vi "Init Name Description.vi"(8 "error in (no error)":errorcluster, 9 "Description":refnum<vi>, 10 "Name":refnum<vi>, 11 "Node Ptr":T1 format="%.0x") -> (0 "error out":errorcluster, 3 "Node Ptr out":T1=18446744073709551615 format="%.0x")   [LabVIEW 2014, in "SLSC configuration System Explorer.lvlib"]
uses:
  SLSC configuration System Explorer.lvlib
  <vilib>/NI Veristand/Custom Device API/Custom Device Item Ref.ctl
  <vilib>/NI Veristand/Custom Device API/Custom Device API.lvlib
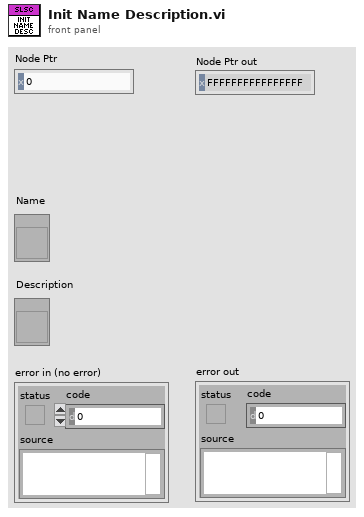
[diagram p1: front panel]
types:
  T1 = typedef "Custom Device API.lvlib/Custom Device Item Ref.ctl" = u64
  T2 = typedef "Custom Device API.lvlib/Custom Device Item Info.ctl" = cluster{"Name":string, "Is Channel":bool, "GUID":string, "Is Waveform":bool}
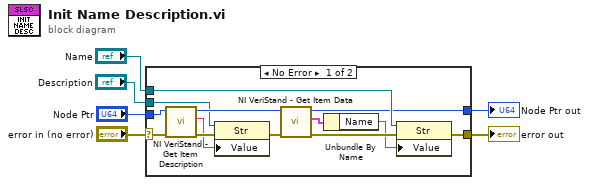
[diagram p0: block diagram]
diagram:
  n1 = case shown="No Error" "error in (no error)" {
    selector: "error in (no error)" -> [w9 w21]
    tunnel: "Node Ptr" -> [w10 w20]
    tunnel: [w7 w20] -> w1
    tunnel: [w8 w21] -> w2
    tunnel: "Description" -> [w12 _]
    tunnel: "Name" -> [w11 _]
    frame No Error {
      n2 = call <vilib>:"NI VeriStand - Get Item Description.vi"("error in (no error)"=w9, "Item Ref in"=w10) -> ("error out"=w19:errorcluster, "Description"=w18:string, "Item Ref out"=w13:T1)  [unwired: 7 out]
      n3 = property class="Str"(reference=w12, error in=w19, "Value"=w18) -> (error out=w16:errorcluster)  [unwired: 1 out]
      n4 = call <vilib>:"NI VeriStand - Get Item Data.vi"("error in (no error)"=w16, "Item Ref in"=w13) -> ("error out"=w15:errorcluster, "Item Info"=w17:T2, "Item Ref out"=w7:T1)  [unwired: 7 out]
      n5 = Unbundle By Name(w17) -> ("Name"=w14:string)
      n6 = property class="Str"(reference=w11, error in=w15, "Value"=w14) -> (error out=w8:errorcluster)  [unwired: 1 out]
    }
    frame Error {
    }
  }
  "error out" <- w2
  "Node Ptr out" <- w1
